vi "ge_ErrorXMLver.vi"(8 "error in":errorcluster, 10 "File Version Number":string) -> (0 "error out":errorcluster)   [LabVIEW 2018]
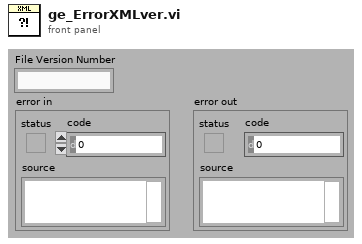
[diagram p1: front panel]
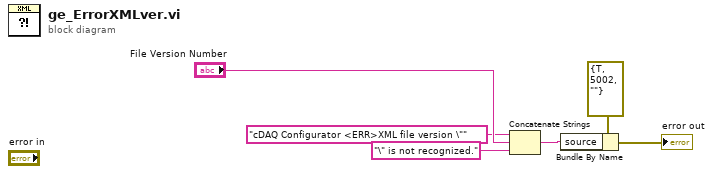
[diagram p0: block diagram]
diagram:
  n1 = Concatenate Strings("cDAQ Configurator <ERR>XML file version \"", "File Version Number", "\" is not recognized." ("string")) -> (w5:string)
  n2 = Bundle By Name(cluster=errorcluster {"status"=TRUE, "code"=5002, "source"=""} ("error out"), "source"=w5) -> (→"error out":errorcluster)
